vi "RageATE_Zip File.vi"(0 "input path":path=path "C:/RageATE Results/REV-B_TETRA_RX-PROD/5_25_2022/REV-B_TETRA_RX-PROD_SN_ RGE2100033_052522-170824_RxCaptureFiles", 11 "error in":errorcluster, 12 "PreserveOrigFolder(t)":bool) -> (3 "NaN/Path/Refnum?":bool, 4 "Generated Zip File":string, 15 "error out":errorcluster)   [LabVIEW 2018]
doc: "This VI will zip up a source directory into a Zip file."
panel:
  # "Select the FOLDER that contains the files to zip.\nThe new zip file will be placed at the same directory level as the folder"
  # "THis vi will take a folder and its contents, zip it and delete the original.\nThe resulting zip file will be at the same directory level and name  as the original\nIf the input path is empty or not valid, the sequence will be skipped and return \"<NotAPath>\""
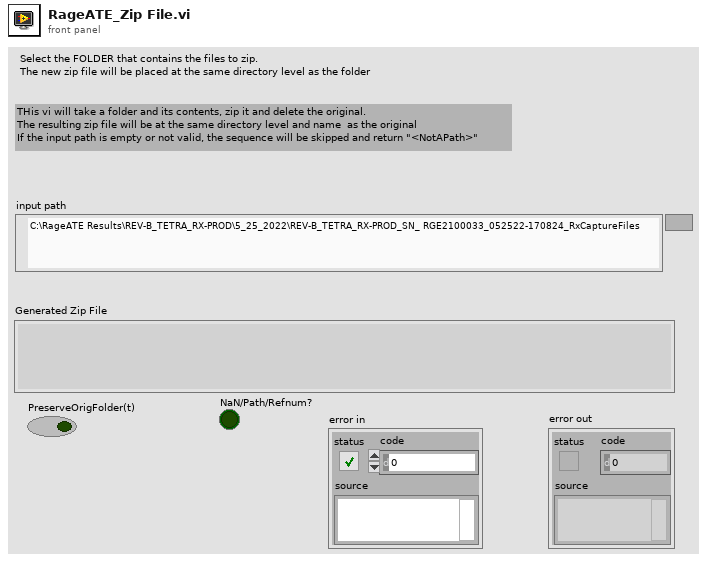
[diagram p1: front panel]
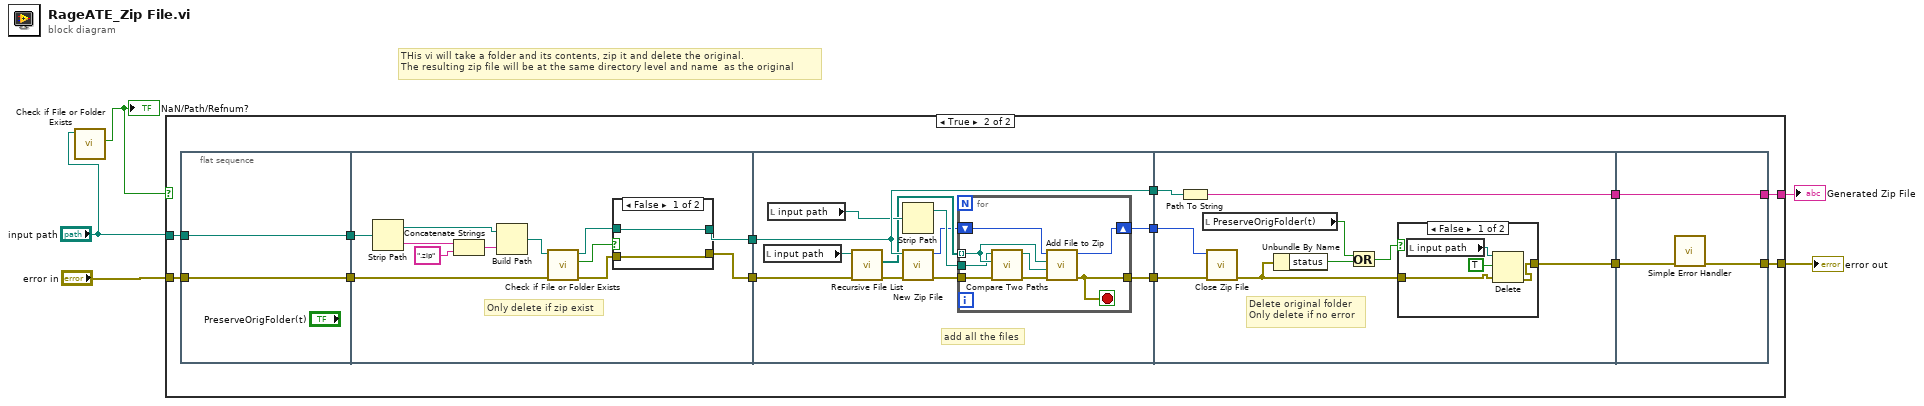
[diagram p0: block diagram]
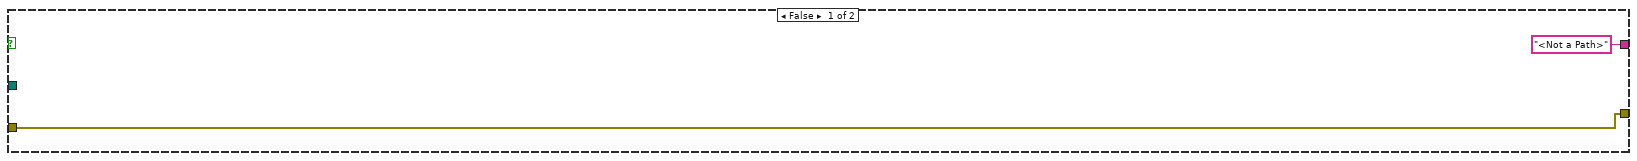
[diagram p2: hidden frame]
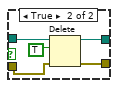
[diagram p3: hidden frame]
diagram:
  # "THis vi will take a folder and its contents, zip it and delete the original.\nThe resulting zip file will be at the same directory level and name  as the original"
  n1 = call <vilib>:"Check if File or Folder Exists.vi"("path"="input path") -> ("file or folder exists?"=w1:bool)  [unwired: 8 in, 2 out]
  "NaN/Path/Refnum?" <- w1
  n2 = case shown="True" w1 {
    tunnel: "input path" -> [_ w11]
    tunnel: [w7 w10] -> w5
    tunnel: "error in" -> [w7 w9]
    tunnel: ["<Not a Path>" w8] -> w3
    frame False {
    }
    frame True {
      n3 = flat-sequence {
        tunnel: [w22] -> w20
        tunnel: [w21] -> w19
        tunnel: w11 -> [w22]
        tunnel: w9 -> [w21]
        tunnel: w20 -> [w29]
        tunnel: [w34] -> w18
        tunnel: w19 -> [w28]
        tunnel: [w24] -> w17
        tunnel: w18 -> [w52]
        tunnel: [w52] -> w16
        tunnel: [w44] -> w15
        tunnel: [w43] -> w14
        tunnel: w17 -> [w42]
        tunnel: w16 -> [w69]
        tunnel: w15 -> [w68]
        tunnel: w14 -> [w67]
        tunnel: [w66] -> w13
        tunnel: [w61] -> w12
        tunnel: w13 -> [w77]
        tunnel: [w76] -> w10
        tunnel: w12 -> [w75]
        tunnel: [w75] -> w8
        frame #0 {
        }
        frame #1 {
          # "Only delete if zip exist"
          n4 = Strip Path(path=w29) -> (stripped path=w30:path, name=w33:string)
          n5 = Concatenate Strings(w33, ".zip" ("string")) -> (w31:string)
          n6 = Build Path(base path=w30, name or relative path=w31) -> (appended path=w27:path)
          n7 = call <vilib>:"Check if File or Folder Exists.vi"("error in (no error)"=w28, "path"=w27) -> ("error out"=w25:errorcluster, "file or folder exists?"=w23:bool, "dup path"=w26:path)  [unwired: 7 in]
          n8 = case shown="False" w23 {
            tunnel: [w36 w41] -> w34
            tunnel: w26 -> [w36 w39]
            tunnel: w25 -> [w35 w38]
            tunnel: [w35 w37] -> w24
            frame False {
            }
            frame True {
              n9 = Delete(path (use dialog)=w39, entire hierarchy (F)=TRUE, error in=w38) -> (deleted path=w41:path, error out=w37:errorcluster)  [unwired: 2 in, 1 out]
            }
          }
        }
        frame #2 {
          # "add all the files"
          n10 = local read "input path"() -> (w51:path)
          n11 = local read "input path"() -> (w50:path)
          n12 = call <vilib>:"Recursive File List.vi"("error in (no error)"=w42, "Folder Path"=w51) -> ("error out"=w47:errorcluster, "All Files in Dir"=w48:path[])  [unwired: 5 in, 3 out]
          n13 = Strip Path(path=w50) -> (stripped path=w49:path)  [unwired: 1 out]
          n14 = call <vilib>:"New Zip File.vi"("error in (no error)"=w47, "target"=w52) -> ("error out"=w46:errorcluster, "zip file out"=w45:i64)  [unwired: 1 in, 3 out]
          n15 = for {
            tunnel: w48 -> [w57] mode=indexing
            tunnel: w46 -> [w54]
            tunnel: [w58] -> w44
            shift-right: [w59] -> w43
            shift-left: w45 -> [w60]
            tunnel: w49 -> [w56]
            stop <- w58 stop-if-true
            n16 = call <vilib>:"Compare Two Paths.vi"("error in (no error)"=w54, "Path 2"=w57, "Path 1"=w56) -> ("error out"=w53:errorcluster, "Relative Path from 1 to 2"=w55:path)  [unwired: 5 in, 2 out]
            n17 = call <vilib>:"Add File to Zip.vi"("error in (no error)"=w53, "destination path in zip"=w55, "source file path"=w57, "zip file in"=w60) -> ("error out"=w58:errorcluster, "zip file out"=w59:i64)  [unwired: 6 out]
          }
        }
        frame #3 {
          # "Delete original folder\nOnly delete if no error"
          n18 = Path To String(path=w69) -> (string=w61:string)
          n19 = local read "PreserveOrigFolder(t)"() -> (w62:bool)
          n20 = call <vilib>:"Close Zip File.vi"("error in (no error)"=w68, "zip file in"=w67) -> ("error out"=w63:errorcluster)  [unwired: 1 in, 4 out]
          n21 = Unbundle By Name(w63) -> ("status"=w64:bool)
          n22 = Or(x=w62, y=w64) -> (x .or. y?=w65:bool)
          n23 = case shown="False" w65 {
            tunnel: [w73 w74] -> w66
            tunnel: w63 -> [w72 w74]
            frame False {
              n24 = local read "input path"() -> (w71:path)
              n25 = Delete(path (use dialog)=w71, entire hierarchy (F)=TRUE, error in=w72) -> (error out=w73:errorcluster)  [unwired: 2 in, 2 out]
            }
            frame True {
            }
          }
        }
        frame #4 {
          n26 = call <vilib>:"Simple Error Handler.vi"("error in (no error)"=w77) -> ("error out"=w76:errorcluster)  [unwired: 1 in, 7 out]
        }
      }
    }
  }
  "error out" <- w5
  "Generated Zip File" <- w3
